vi "Initialize Convert Buffers.vi"(8 "error in":errorcluster, 10 "Group Configurations":refnum<class "Group Configuration.lvclass">[](array[class]), 11 "Type Converter":refnum<class "Default Buffer Converter.lvclass">) -> (0 "error out":errorcluster, 3 "Type Converter out":refnum<class "Default Buffer Converter.lvclass">)   [LabVIEW 2021, in "DSF Core.lvlib" / "Default Buffer Converter.lvclass"]
uses:
  Default Buffer Converter.lvclass
  Classes/Configuration/Core/Group/Group Configuration.lvclass
  Default Buffer Converter.lvclass/Default Buffer Converter.ctl
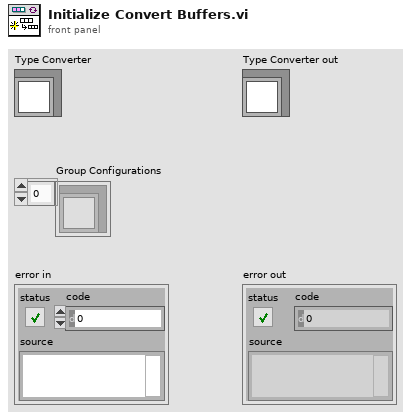
[diagram p1: front panel]
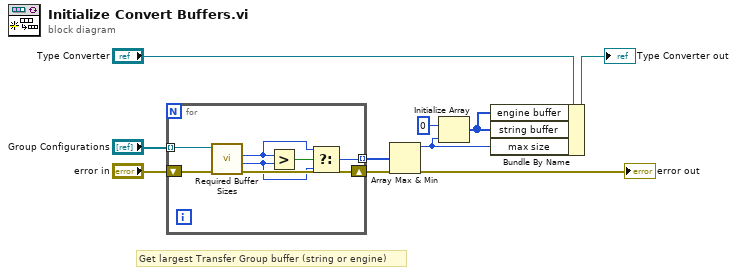
[diagram p0: block diagram]
diagram:
  # "Get largest Transfer Group buffer (string or engine)"
  n1 = for {
    tunnel: "Group Configurations" -> [w14] mode=indexing
    tunnel: [w15] -> w9 mode=indexing
    shift-right: [w11] -> w4
    shift-left: "error in" -> [w13]
    n2 = call-dynamic "Required Buffer Sizes.vi"("error in (no error)"=w13, "Group Configuration in"=w14) -> ("error out"=w11:errorcluster, "string size"=w10:u64, "engine size"=w12:u64)  [unwired: 6 in, 1 out]
    n3 = Greater?(x=w12, y=w10) -> (0:w16:bool)
    n4 = Select(t=w12, s=w16, f=w10) -> (s? t:f=w15:u64)
  }
  "error out" <- w4
  n5 = Array Max & Min(array=w9) -> (max value=w6:u64)  [unwired: 3 out]
  n6 = Initialize Array(u8 0, w6) -> (w5:u8[])
  n7 = Bundle By Name(cluster="Type Converter", "engine buffer"=w5, "string buffer"=w5, "max size"=w6) -> (→"Type Converter out":refnum<class "Default Buffer Converter.lvclass">)
